vi "createControls.vi"(8 "error in (no error)":errorcluster, 10 "libraryInfo":T1, 11 "Enumeration in":refnum<class "Enumeration.lvclass">) -> (0 "error out":errorcluster, 3 "Enumeration out":refnum<class "Enumeration.lvclass">)   [LabVIEW 2016, in "Enumeration.lvclass"]
uses:
  Enumeration.lvclass
  Typedefs/LibraryInfo.ctl
  Enumeration.lvclass/Enumeration.ctl
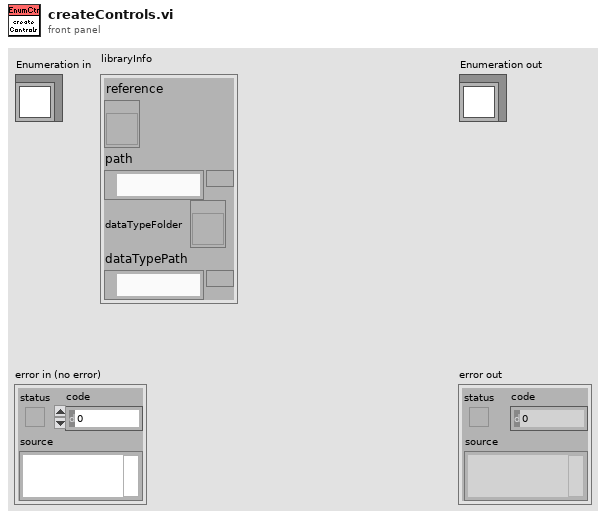
[diagram p1: front panel]
types:
  T1 = typedef "LibraryInfo.ctl" = cluster{"reference":refnum<vi>, "path":path, "dataTypeFolder":refnum<vi>, "dataTypePath":path}
  T2 = enum32{"not a control VI", "control", "typedef", "strict typedef"}
  T3 = enum32{"invalid VI type", "Standard VI", "Control VI", "Global VI", "Polymorphic VI", "Configuration VI", "SubSystem", "Facade VI", "Method VI", "Statechart Diagram VI"}
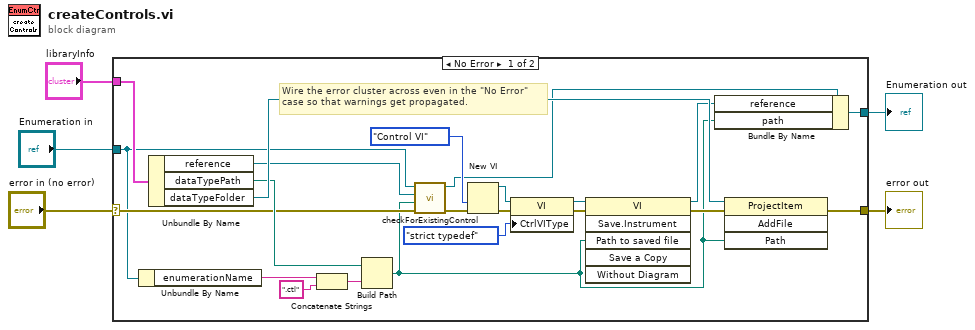
[diagram p0: block diagram]
diagram:
  n1 = case shown="No Error" "error in (no error)" {
    selector: "error in (no error)" -> [w11 w29]
    tunnel: [w10 w29] -> w4
    tunnel: [w8 w28] -> w2
    tunnel: "Enumeration in" -> [w9 w28]
    tunnel: "libraryInfo" -> [w14 _]
    frame No Error {
      # "Wire the error cluster across even in the \"No Error\"\ncase so that warnings get propagated."
      n2 = Unbundle By Name(w9) -> ("enumerationName"=w20:string)
      n3 = Unbundle By Name(w14) -> ("reference"=w7:refnum<vi>, "dataTypePath"=w21:path, "dataTypeFolder"=w27:refnum<vi>)
      n4 = Concatenate Strings(w20, ".ctl" ("string")) -> (w17:string)
      n5 = Build Path(base path=w21, name or relative path=w17) -> (appended path=w6:path)
      n6 = call "checkForExistingControl.vi"("error in (no error)"=w11, "controlPath"=w6, "libraryRef"=w7, "Enumeration in"=w9) -> ("error out"=w12:errorcluster, "Enumeration out"=w13:refnum<class "Enumeration.lvclass">)  [unwired: 6 in]
      n7 = New VI(8:w12, 9:T3."Control VI" ("vi type (standard vi)")) -> (0:w24:errorcluster, 3:w18:refnum<vi>)  [unwired: 5 in]
      n8 = property class="VI"(reference=w18, error in=w24, "CtrlVIType"=T2."strict typedef" ("Control VI Type")) -> (reference out=w26:refnum<vi>, error out=w25:errorcluster)
      n9 = invoke class="VI" method="Save.Instrument"(reference=w26, error in=w25, "Path to saved file"=w6) -> (reference out=w22:refnum<vi>, error out=w23:errorcluster)  [unwired: 3 in, 4 out]
      n10 = Bundle By Name(cluster=w13, "reference"=w22, "path"=w6) -> (w8:refnum<class "Enumeration.lvclass">)
      n11 = invoke class="ProjectItem" method="AddFile"(reference=w27, error in=w23, "Path"=w6) -> (error out=w10:errorcluster)  [unwired: 1 in, 3 out]
    }
    frame Error {
    }
  }
  "error out" <- w4
  "Enumeration out" <- w2
